vi "Camera Begin.vi"   [LabVIEW 2013]
uses:
  <vilib>/Rock Robotics/SystemInterfaces/DIO/FPGA_DIOPWMChannel.ctl
  <vilib>/Rock Robotics/SystemInterfaces/Typedef/FPGA_TypedefDigitalModule.ctl
types:
  T1 = typedef "FPGA_TypedefDigitalModule.ctl" = enum16{"Digital Module 1", "Digital Module 2"}
  T2 = typedef "FPGA_DIOPWMChannel.ctl" = enum8{"PWM 1", "PWM 2", "PWM 3", "PWM 4", "PWM 5", "PWM 6", "PWM 7", "PWM 8", "PWM 9", "PWM 10", "Invalid"}
  T3 = typedef "WPI_ServoDeviceRef.ctl" = cluster{"DeviceStatus":errorcluster, "Digital Module":T1, "PWM Channel":T2, "DeadBand":T4}
  T4 = typedef "WPI_PWMDeadband.ctl" = cluster{"Name":string, "maxPositivePwm":i32, "minPositivePwm":i32, "centerPwm":i32, "maxNegativePwm":i32, "minNegativePwm":i32, "angularRange":u16}
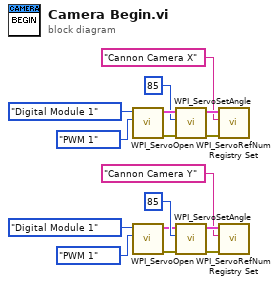
[diagram p0: block diagram]
diagram:
  n1 = call <vilib>:"WPI_ServoOpen.vi"("PWM Channel"=FPGA_DIOPWMChannel."PWM 1", "Digital Module (Module 1)"=FPGA_TypedefDigitalModule."Digital Module 1") -> ("error out"=w16:errorcluster, "ServoDeviceRef"=w15:T3)  [unwired: 8 in]
  n2 = call <vilib>:"WPI_ServoOpen.vi"("PWM Channel"=FPGA_DIOPWMChannel."PWM 1", "Digital Module (Module 1)"=FPGA_TypedefDigitalModule."Digital Module 1") -> ("error out"=w3:errorcluster, "ServoDeviceRef"=w4:T3)  [unwired: 8 in]
  n3 = call <vilib>:"WPI_ServoSetAngle.vi"("error in (no error)"=w16, "Angle"=85, "ServoDeviceRef"=w15) -> ("error out"=w14:errorcluster, "ServoDeviceRef"=w13:T3)  [unwired: 7 in]
  n4 = call <vilib>:"WPI_ServoSetAngle.vi"("error in (no error)"=w3, "Angle"=85, "ServoDeviceRef"=w4) -> ("error out"=w5:errorcluster, "ServoDeviceRef"=w6:T3)  [unwired: 7 in]
  n5 = call <vilib>:"WPI_ServoRefNum Registry Set.vi"("error in (no error)"=w14, "refnum name"="Cannon Camera X", "ServoDeviceRef"=w13) -> ()  [unwired: 7 in, 2 out]
  n6 = call <vilib>:"WPI_ServoRefNum Registry Set.vi"("error in (no error)"=w5, "refnum name"="Cannon Camera Y", "ServoDeviceRef"=w6) -> ()  [unwired: 7 in, 2 out]
